vi "判斷式簡易版.vi"(1 "Vc":dbl, 2 "Va":dbl, 3 "H":dbl, 4 "S0":dbl) -> (0 "result":bool)   [LabVIEW 2014]
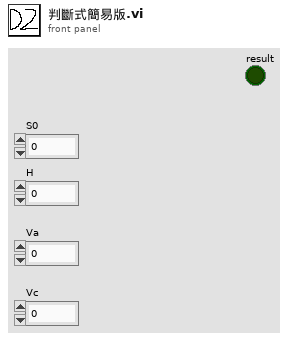
[diagram p1: front panel]
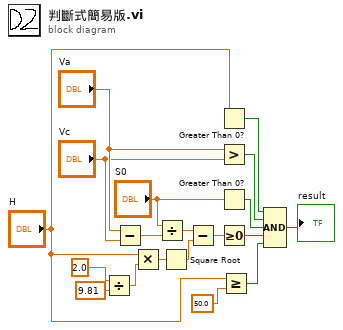
[diagram p0: block diagram]
diagram:
  n1 = Divide(x=2.0, y=9.81) -> (x/y=w12:dbl)
  n2 = Subtract(x="Va", y="Vc") -> (x-y=w15:dbl)
  n3 = Multiply(x="H", y=w12) -> (x*y=w11:dbl)
  n4 = Divide(x="S0", y=w15) -> (x/y=w10:dbl)
  n5 = Square Root(x=w11) -> (sqrt(x)=w9:dbl)
  n6 = Subtract(x=w10, y=w9) -> (x-y=w5:dbl)
  n7 = Greater Than 0?(x="H") -> (x > 0?=w19:bool)
  n8 = Greater?(x="Va", y="Vc") -> (0:w18:bool)
  n9 = Greater Than 0?(x="S0") -> (x > 0?=w17:bool)
  n10 = Greater Or Equal To 0?(x=w5) -> (x >= 0?=w4:bool)
  n11 = Greater Or Equal?(x="H", y=50.0) -> (x >= y?=w2:bool)
  n12 = Compound Arithmetic op=AND(w19, w18, w17, w4, w2) -> (→"result":bool)
